vi "FeedbackDecode_RunProgram_PSExec.vi"(1 "ProgramInput":string, 2 "Program":path=path "D:/RemoteRepo/RippleEMG.exe", 3 "ComputerName":string="PNIMatlab", 4 "Mode":enum16{"Start", "Stop"}(ring)) -> (0 "standard output":string)   [LabVIEW 2020]
panel:
  out "standard error 2":string
  out "ProgStr":string="D:\\RemoteRepo\\RippleEMG.exe"
  out "standard error":string
  out "Result":string
  out "ProcessId":string
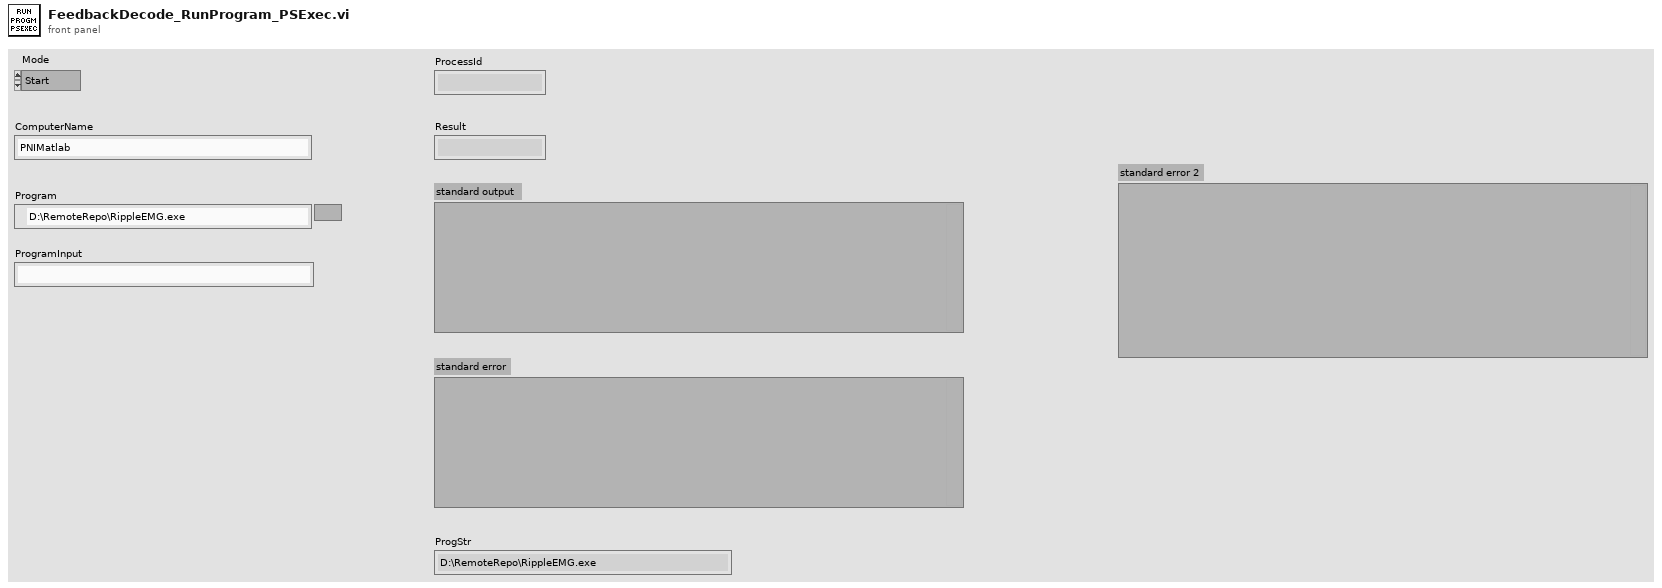
[diagram p1: front panel]
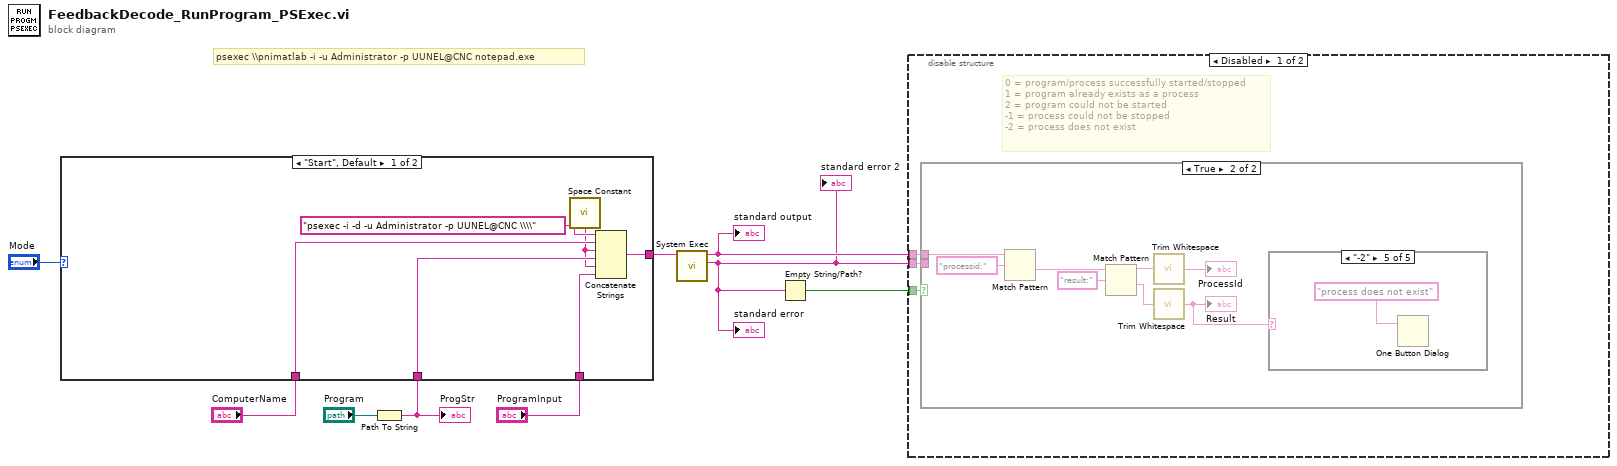
[diagram p0: block diagram]
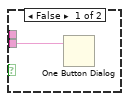
[diagram p2: hidden frame]
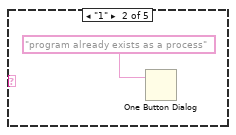
[diagram p4: hidden frame]
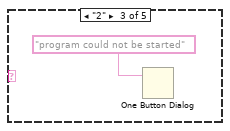
[diagram p5: hidden frame]
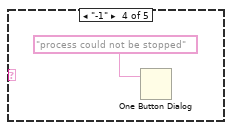
[diagram p6: hidden frame]
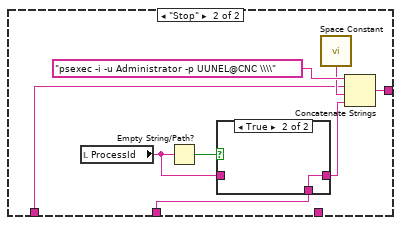
[diagram p8: hidden frame]
diagram:
  # "psexec \\\\pnimatlab -i -u Administrator -p UUNEL@CNC notepad.exe"
  n1 = Path To String(path="Program") -> (string=w2:string)
  "ProgStr" <- w2
  n2 = case shown="\"Start\", Default" "Mode" {
    tunnel: [w14 w21] -> w9
    tunnel: "ComputerName" -> [w13 w17]
    tunnel: w2 -> [w12 w16]
    tunnel: "ProgramInput" -> [w10 _]
    frame "Start", Default {
      n3 = call <vilib>:"Space Constant.vi"() -> ("String"=w11:string)
      n4 = Concatenate Strings("psexec -i -d -u Administrator -p UUNEL@CNC \\\\" ("command line"), w13, w11, w12, w11, w10) -> (w14:string)
    }
    frame "Stop" {
      n5 = local read "ProcessId"() -> (w19:string)
      n6 = Empty String/Path?(string/path=w19) -> (empty?=w20:bool)
      n7 = case shown="True" w20 {
        tunnel: w19 -> [w24 _]
        tunnel: [w24 w25] -> w18
        tunnel: w16 -> [_ w25]
        frame False {
        }
        frame True {
        }
      }
      n8 = call <vilib>:"Space Constant.vi"() -> ("String"=w22:string)
      n9 = Concatenate Strings("psexec -i -u Administrator -p UUNEL@CNC \\\\" ("command line"), w17, w22, w18) -> (w21:string)
    }
  }
  n10 = call <vilib>:"System Exec.vi"("command line"=w9) -> ("standard error"=w5:string, "standard output"=w8:string)  [unwired: 7 in, 2 out]
  "standard output" <- w8
  "standard error" <- w5
  "standard error 2" <- w5
  n11 = Empty String/Path?(string/path=w5) -> (empty?=w6:bool)
  n12 = disable-structure shown="Disabled" {
    disable-tunnel: w8 -> [w28 _]
    disable-tunnel: w6 -> [w27 _]
    disable-tunnel: w5 -> [w26 _]
    frame Disabled {
      # "0 = program/process successfully started/stopped\n1 = program already exists as a process\n2 = program could not be started\n-1 = process could not be stopped\n-2 = process does not exist"
      n13 = case shown="True" w27 {
        tunnel: w28 -> [_ w37]
        tunnel: w26 -> [w29 _]
        frame False {
          n14 = One Button Dialog(message=w29) -> ()  [unwired: 1 in, 1 out]
        }
        frame True {
          n15 = Match Pattern(string=w37, regular expression="processid:") -> (after substring=w35:string)  [unwired: 1 in, 3 out]
          n16 = Match Pattern(string=w35, regular expression="result:") -> (before substring=w33:string, after substring=w32:string)  [unwired: 1 in, 2 out]
          n17 = call <vilib>:"Trim Whitespace.vi"("string"=w33) -> ("trimmed string"=→"ProcessId":string)  [unwired: 1 in]
          n18 = call <vilib>:"Trim Whitespace.vi"("string"=w32) -> ("trimmed string"=w31:string)  [unwired: 1 in]
          "Result" <- w31
          n19 = case shown="\"-2\"" w31 {
            frame "0", Default {
            }
            frame "1" {
              n20 = One Button Dialog(message="program already exists as a process") -> ()  [unwired: 1 in, 1 out]
            }
            frame "2" {
              n21 = One Button Dialog(message="program could not be started") -> ()  [unwired: 1 in, 1 out]
            }
            frame "-1" {
              n22 = One Button Dialog(message="process could not be stopped") -> ()  [unwired: 1 in, 1 out]
            }
            frame "-2" {
              n23 = One Button Dialog(message="process does not exist") -> ()  [unwired: 1 in, 1 out]
            }
          }
        }
      }
    }
    frame Enabled {
    }
  }
